vi "Server_Main.vi"() -> ()   [LabVIEW 2018]
uses:
  <vilib>/MediaMongrels Ltd/WebSockets/WebSockets/WebSocket Server/WebSocket Server.lvclass
  <vilib>/Platform/browser.llb/Open URL in Default Browser (string).vi
panel:
  out "Connected":bool
  in  "connect":bool
  in  "File:":u16(ring) items=["01_2_Script.docx", "<none>"]
  in  "web":bool
  out "Data":string="I am looking forward\nto reading this on\nmy phone"
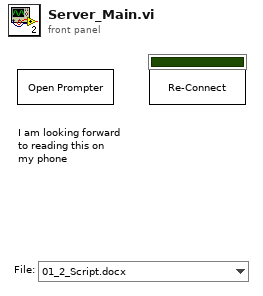
[diagram p1: front panel]
types:
  T1 = cluster{"index":i32, "Chunks":string[], "WebSocket":refnum<class "WebSocket Server.lvclass">, "DocPaths":string[], "DocNames":string[], "Con":bool}
  T2 = enum32{"Invalid", "Standard", "Closed", "Hidden", "Minimized", "Maximized"}
  T3 = enum32{"invalid app kind", "Development System", "Run Time System", "Student Edition", "Embedded LabVIEW", "Evaluation", "Custom"}
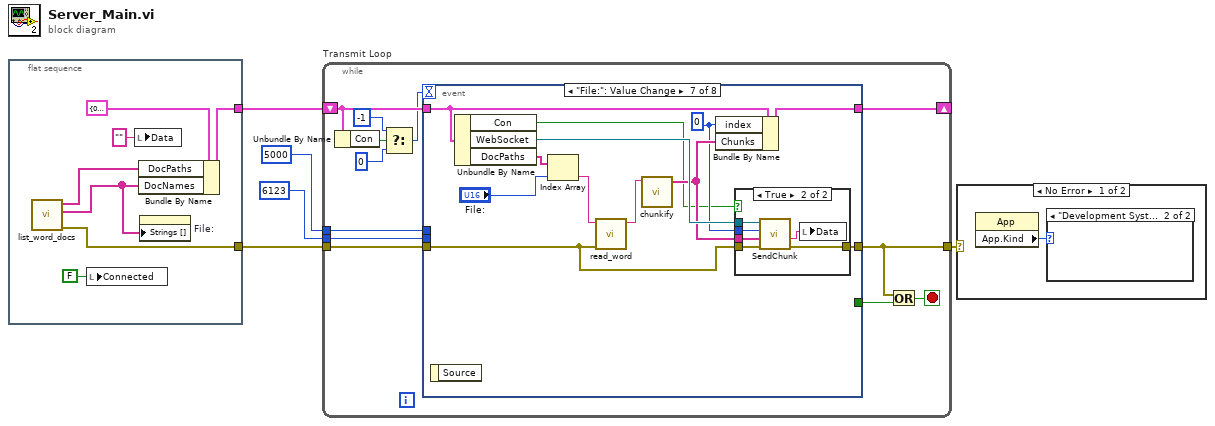
[diagram p0: block diagram]
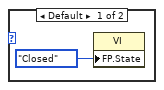
[diagram p2: hidden frame]
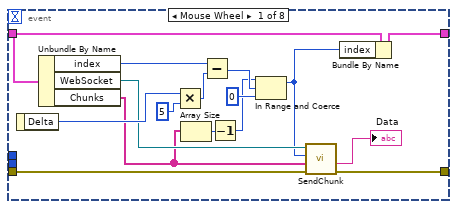
[diagram p4: hidden frame]
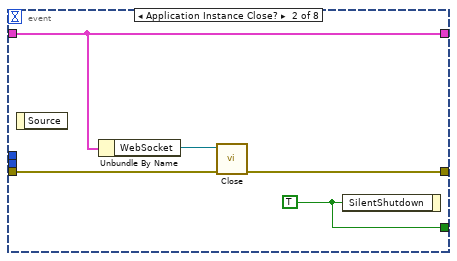
[diagram p5: hidden frame]
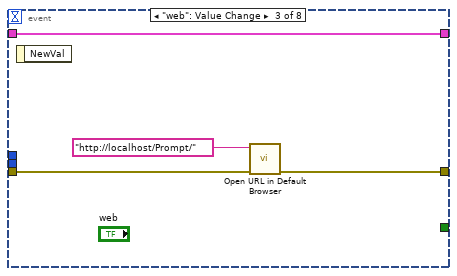
[diagram p6: hidden frame]
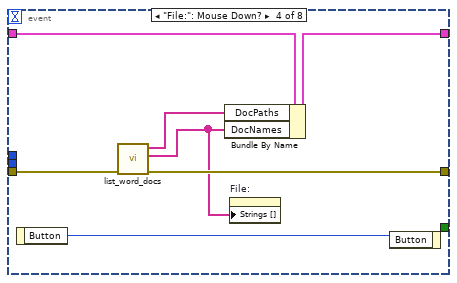
[diagram p7: hidden frame]
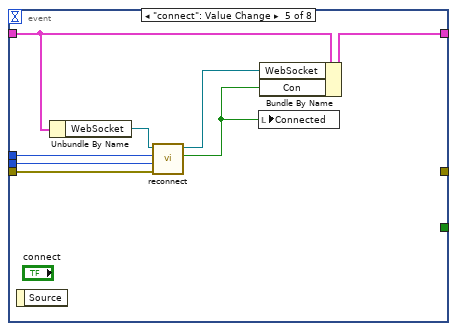
[diagram p8: hidden frame]
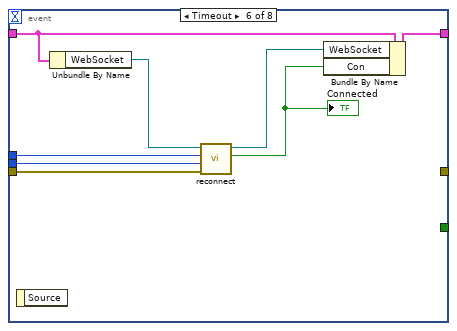
[diagram p9: hidden frame]
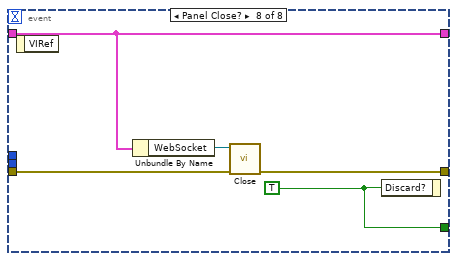
[diagram p11: hidden frame]
diagram:
  n1 = flat-sequence {
    tunnel: [w9] -> w3
    tunnel: [w8] -> w2
    frame #0 {
      n2 = call "list_word_docs.vi"() -> ("error out"=w8:errorcluster, "DocumentNames"=w12:string[], "DocumentPaths"=w11:string[])  [unwired: 9 in]
      n3 = local write "Connected"(FALSE ("Connected")) -> ()
      n4 = local write "Data"("" ("Data")) -> ()
      n5 = Bundle By Name(cluster=T1 {"index"=0, "Chunks"=[], "WebSocket"=refnum, "DocPaths"=[], "DocNames"=[], "Con"=FALSE}, "DocPaths"=w11, "DocNames"=w12) -> (w9:T1)
      n6 = property on="File:" class="Ring (strict)"("Strings []"=w12) -> ()  [unwired: 2 in, 2 out]
    }
  }
  n7 = while "Transmit Loop" {
    tunnel: w2 -> [w24]
    shift-right: [w21] -> _
    shift-left: w3 -> [w18]
    tunnel: 5000 ("timeout ms (25000)") -> [w20]
    tunnel: u16 6123 ("port") -> [w19]
    tunnel: [w13] -> w1
    stop <- w22 stop-if-true
    n8 = Unbundle By Name(w18) -> ("Con"=w17:bool)
    n9 = Select(t=-1, s=w17, f=0) -> (s? t:f=w14:i32)
    n10 = event shown="[6] \"File:\": Value Change" {
      selector: _ -> [_ _ _ _ _ _ _ _]
      dyn-events: _ -> [_ _ _ _ _ _ _ _]
      timeout: w14 -> [_ _ _ _ _ _ _ _]
      tunnel: [_ w43 _ _ _ _ _ w96] -> w23
      tunnel: [w40 w45 w49 w54 _ _ w74 w95] -> w13
      tunnel: w24 -> [w39 w44 w48 w55 w63 w71 w75 w94]
      tunnel: w18 -> [w35 w42 w46 w56 w62 w70 w84 w93]
      tunnel: [w33 w42 w46 w53 w61 w69 w83 w93] -> w21
      tunnel: w20 -> [_ _ _ _ w59 w67 _ _]
      tunnel: w19 -> [_ _ _ _ w58 w66 _ _]
      event Mouse Wheel {
        n11 = event-data() -> ("Delta"=w38:i32)  [unwired: 1 in]
        n12 = Unbundle By Name(w35) -> ("index"=w34:i32, "WebSocket"=w32:refnum<class "WebSocket Server.lvclass">, "Chunks"=w30:string[])
        n13 = Multiply(x=w38, y=5) -> (x*y=w37:i32)
        n14 = Array Size(array=w30) -> (size(s)=w29:i32)
        n15 = Subtract(x=w34, y=w37) -> (x-y=w26:i32)
        n16 = Decrement(x=w29) -> (x-1=w25:i32)
        n17 = In Range and Coerce(upper limit=w25, x=w26, lower limit=0) -> (coerced(x)=w27:i32)  [unwired: 1 out]
        n18 = call "SendChunk.vi"("error in (no error)"=w39, "Chunks"=w30, "index"=w27, "WebSocket Server in"=w32) -> ("error out"=w40:errorcluster, "Chunk"=→"Data":string)  [unwired: 5 in, 1 out]
        n19 = Bundle By Name(cluster=w35, "index"=w27) -> (w33:T1)
      }
      event Application Instance Close? {
        w43 = TRUE ("SilentShutdown")
        n20 = event-data() -> ()  [unwired: 1 in, 1 out]
        n21 = Unbundle By Name(w42) -> ("WebSocket"=w41:refnum<class "WebSocket Server.lvclass">)
        n22 = call-dynamic "Close.vi"("error in (no error)"=w44, "WebSocket in"=w41) -> ("error out"=w45:errorcluster)  [unwired: 9 in]
        n23 = event-data("SilentShutdown"=w43) -> ()  [unwired: 1 in, 1 out]
      }
      event "web": Value Change {
        n24 = event-data() -> ()  [unwired: 1 in, 1 out]
        n25 = call-poly <vilib>:"Open URL in Default Browser.vi"("error in (no error)"=w48, "URL"="http://localhost/Prompt/") -> ("error out"=w49:errorcluster)  [unwired: 4 in, 1 out]
      }
      event "File:": Mouse Down? {
        n26 = event-data() -> ("Button"=w50:u16)  [unwired: 1 in]
        n27 = call "list_word_docs.vi"("error in (no error)"=w55) -> ("error out"=w54:errorcluster, "DocumentNames"=w51:string[], "DocumentPaths"=w52:string[])  [unwired: 8 in]
        n28 = Bundle By Name(cluster=w56, "DocPaths"=w52, "DocNames"=w51) -> (w53:T1)
        n29 = property on="File:" class="Ring (strict)"("Strings []"=w51) -> ()  [unwired: 2 in, 2 out]
        n30 = event-data("Button"=w50) -> ()  [unwired: 1 in, 1 out]
      }
      event "connect": Value Change {
        n31 = event-data() -> ()  [unwired: 1 in, 1 out]
        n32 = Unbundle By Name(w62) -> ("WebSocket"=w64:refnum<class "WebSocket Server.lvclass">)
        n33 = call "reconnect.vi"("error in (no error)"=w63, "port"=w58, "timeout ms (25000)"=w59, "WebSocket in"=w64) -> ("Connected"=w57:bool, "WebSocket out"=w60:refnum<class "WebSocket Server.lvclass">)  [unwired: 5 in, 1 out]
        n34 = local write "Connected"(w57) -> ()
        n35 = Bundle By Name(cluster=w62, "WebSocket"=w60, "Con"=w57) -> (w61:T1)
      }
      event Timeout {
        n36 = event-data() -> ()  [unwired: 1 in, 1 out]
        n37 = Unbundle By Name(w70) -> ("WebSocket"=w72:refnum<class "WebSocket Server.lvclass">)
        n38 = call "reconnect.vi"("error in (no error)"=w71, "port"=w66, "timeout ms (25000)"=w67, "WebSocket in"=w72) -> ("Connected"=w65:bool, "WebSocket out"=w68:refnum<class "WebSocket Server.lvclass">)  [unwired: 5 in, 1 out]
        "Connected" <- w65
        n39 = Bundle By Name(cluster=w70, "WebSocket"=w68, "Con"=w65) -> (w69:T1)
      }
      event "File:": Value Change {
        w76 = 0 ("index")
        n40 = event-data() -> ()  [unwired: 1 in, 1 out]
        n41 = Unbundle By Name(w84) -> ("Con"=w73:bool, "WebSocket"=w78:refnum<class "WebSocket Server.lvclass">, "DocPaths"=w82:string[])
        n42 = Index Array(array=w82, index="File:") -> (element=w80:string)
        n43 = call "read_word.vi"("error in (no error)"=w75, "FilePath"=w80) -> ("Text"=w79:string)  [unwired: 9 in]
        n44 = call "chunkify.vi"("String"=w79) -> ("Chunks"=w77:string[])  [unwired: 10 in]
        n45 = Bundle By Name(cluster=w84, "index"=w76, "Chunks"=w77) -> (w83:T1)
        n46 = case shown="True" w73 {
          tunnel: w78 -> [_ w91]
          tunnel: w77 -> [_ w90]
          tunnel: w76 -> [_ w89]
          tunnel: w75 -> [w85 w88]
          tunnel: [w85 w87] -> w74
          frame False {
          }
          frame True {
            n47 = call "SendChunk.vi"("error in (no error)"=w88, "Chunks"=w90, "index"=w89, "WebSocket Server in"=w91) -> ("error out"=w87:errorcluster, "Chunk"=w86:string)  [unwired: 5 in, 1 out]
            n48 = local write "Data"(w86) -> ()
          }
        }
      }
      event Panel Close? {
        w96 = TRUE ("Discard?")
        n49 = event-data() -> ()  [unwired: 1 in, 1 out]
        n50 = Unbundle By Name(w93) -> ("WebSocket"=w92:refnum<class "WebSocket Server.lvclass">)
        n51 = call-dynamic "Close.vi"("error in (no error)"=w94, "WebSocket in"=w92) -> ("error out"=w95:errorcluster)  [unwired: 9 in]
        n52 = event-data("Discard?"=w96) -> ()  [unwired: 1 in, 1 out]
      }
    }
    n53 = Or(x=w13, y=w23) -> (x .or. y?=w22:bool)
  }
  n54 = case shown="No Error" w1 {
    frame No Error {
      n55 = property class="App"() -> ("App.Kind"=w97:T3)  [unwired: 2 in, 2 out]
      n56 = case shown="\"Development System\"" w97 {
        frame Default {
          n57 = property class="VI"("FP.State"=T2."Closed" ("Front Panel Window:State")) -> ()  [unwired: 2 in, 2 out]
        }
        frame "Development System" {
        }
      }
    }
    frame Error {
    }
  }
